vi "RS485ReadNormal2.vi"() -> ()   [LabVIEW 2016]
uses:
  <vilib>/Instr/_visa.llb/VISA Configure Serial Port (Instr).vi
panel:
  out "Measurement":dbl[](array[numeric])
  out "Time Interval":dbl[](array[numeric])
  in  "VISA resource name":refnum<visa-resource-name>="COM4"
  in  "flow control":u16(ring) items=["None"=0, "XON/XOFF"=1, "RTS/CTS"=2, "DTR/DSR"=4]
  in  "stop bits":u16(ring)=10 items=["1"=10, "1.5"=15, "2.0"=20]
  in  "parity":u16(ring)=2 items=["None", "Odd", "Even", "Mark", "Space"]
  in  "data bits":u16=8 min=5 max=8 step=1
  in  "baud rate":u32=1500000
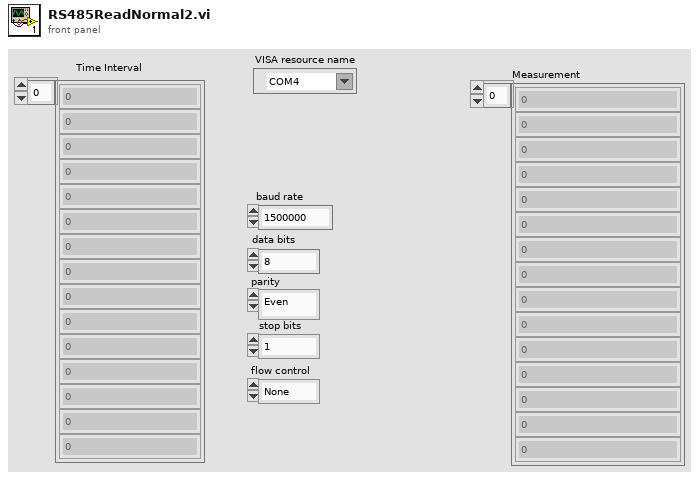
[diagram p1: front panel]
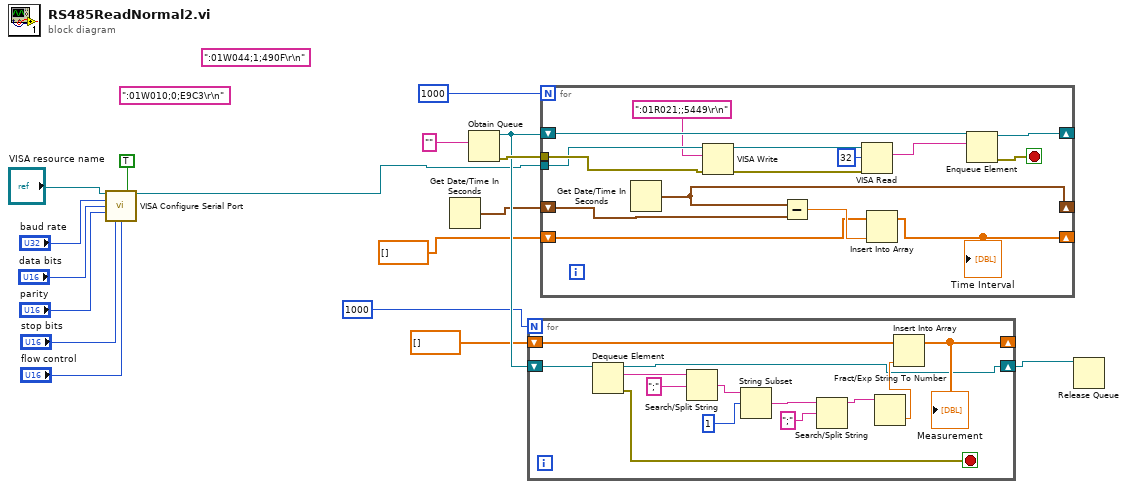
[diagram p0: block diagram]
diagram:
  (unwired) ":01W010;0;E9C3\r\n" ("write buffer")
  (unwired) ":01W044;1;490F\r\n" ("write buffer")
  n1 = call-poly "VISA Configure Serial Port"("VISA resource name"="VISA resource name", "Enable Termination\nChar (T)"=TRUE, "baud rate (9600)"="baud rate", "data bits (8)"="data bits", "parity (0:none)"="parity", "stop bits (10: 1 bit)"="stop bits", "flow control (0:none)"="flow control") -> ("VISA resource name out"=w1:refnum<visa-resource-name>)  [unwired: 7 in, 1 out]
  n2 = Get Date/Time In Seconds() -> (seconds since 1Jan1904=w6:timestamp)
  n3 = Obtain Queue(element data type="" ("write buffer")) -> (queue out=w7:refnum<queue>, error out=w8:errorcluster)  [unwired: 4 in, 1 out]
  n4 = for {
    N: 1000 -> [_]
    shift-right: [w18] -> w2
    shift-left: w7 -> [w30]
    shift-right: [w20] -> _
    shift-left: dbl[] [] -> [w21]
    stop <- w22 stop-if-true
    n5 = Dequeue Element(queue=w30) -> (queue out=w18:refnum<queue>, element=w23:string, error out=w22:errorcluster)  [unwired: 2 in, 1 out]
    n6 = Search/Split String(string=w23, search string/char (-)=";") -> (match + rest of string=w29:string)  [unwired: 1 in, 2 out]
    n7 = String Subset(string=w29, offset (0)=1) -> (substring=w26:string)  [unwired: 1 in]
    n8 = Search/Split String(string=w26, search string/char (-)=";") -> (substring before match=w28:string)  [unwired: 1 in, 2 out]
    n9 = Fract/Exp String To Number(string=w28) -> (number=w19:dbl)  [unwired: 3 in, 1 out]
    n10 = Insert Into Array(array=w21, new element=w19) -> (w20:dbl[])  [unwired: 1 in]
    "Measurement" <- w20
  }
  n11 = for {
    N: 1000 -> [_]
    tunnel: w1 -> [w32]
    tunnel: w8 -> [w35]
    shift-right: [w44] -> _
    shift-left: w7 -> [w43]
    shift-right: [w40] -> _
    shift-left: w6 -> [w41]
    shift-right: [w37] -> _
    shift-left: dbl[] [] -> [w38]
    stop <- w42 stop-if-true
    n12 = Get Date/Time In Seconds() -> (seconds since 1Jan1904=w40:timestamp)
    n13 = VISA Write(VISA resource name=w32, write buffer=":01R021;;5449\r\n", error in (no error)=w35) -> (VISA resource name out=w33:refnum<visa-resource-name>, error out=w34:errorcluster)  [unwired: 1 out]
    n14 = Subtract(x=w40, y=w41) -> (x-y=w39:dbl)
    n15 = VISA Read(VISA resource name=w33, byte count=u32 32, error in (no error)=w34) -> (read buffer=w45:string)  [unwired: 3 out]
    n16 = Insert Into Array(array=w38, new element=w39) -> (w37:dbl[])  [unwired: 1 in]
    "Time Interval" <- w37
    n17 = Enqueue Element(queue=w43, element=w45) -> (queue out=w44:refnum<queue>, error out=w42:errorcluster)  [unwired: 2 in, 1 out]
  }
  n18 = Release Queue(queue=w2) -> ()  [unwired: 2 in, 3 out]
